vi "Get Number Photon Counting Divisions.vi"(11 "noOfDivisions":u32) -> (2 "function return":u32, 3 "noOfDivisions out":u32)   [LabVIEW 2018, in "AndorSDK.lvlib"]
doc: "EXPNETTYPE unsigned int WINAPI GetNumberPhotonCountingDivisions(at_u32 * noOfDivisions);"
uses:
  AndorSDK.lvlib
  ATMCD32D.dll
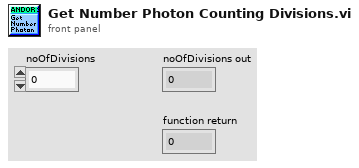
[diagram p1: front panel]
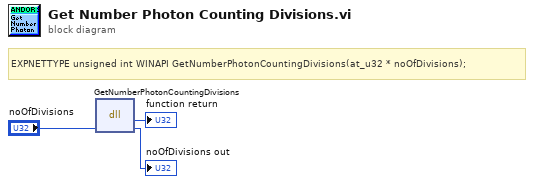
[diagram p0: block diagram]
diagram:
  # "EXPNETTYPE unsigned int WINAPI GetNumberPhotonCountingDivisions(at_u32 * noOfDivisions);"
  n1 = dll-call lib="PTH2babs E\nPersönliches02 - Arbeit03-HiwijobsLabviewCodelibANDOR\tAndor SDK\nATMCD32D.*" fn="GetNumberPhotonCountingDivisions"("noOfDivisions"="noOfDivisions") -> (→"function return":u32, "noOfDivisions"=→"noOfDivisions out":u32)  [unwired: 3 in, 2 out]
